vi "Instrumento_caracterizacion_3.vi"() -> ()   [LabVIEW 2009]
uses:
  <vilib>/Analysis/NI_AALBase.lvlib
panel:
  in  "Nombre de archivo":string="In1"
  in  "Activate switches 2":bool
  out "?":bool
  in  "Seleción método":bool
  in  "Ángulos de elementos ópticos:\nL2_in        L4_in     L4_out  P__out":dbl[](array[numeric])=[0.0, 0.0, 0.0, 0.0]
  in  "Amp vs ng":bool
  in  "fas vs ng":bool
  in  "Directorio scripts matlab 2":path=path "C:/Users/franjas/Documents/rutinas-calibracion-slm"
  in  "Exit live":bool
  in  "Capture":bool
  in  "stop":bool
  in  "File to load":path
  in  "File to save":path
  in  "VCD Properties":bool
  in  "Save properties":bool
  in  "Load properties":bool
  in  "Configurar para franjas":bool
  out "Histogram Graph":T1(graph)
  in  "Run live preview":bool
  out "Live Picture":picture
  out "Video formats":string[](array[string])
  out "Devices":string[](array[string])
  in  "ICImagingControl":refnum<k7>(container)
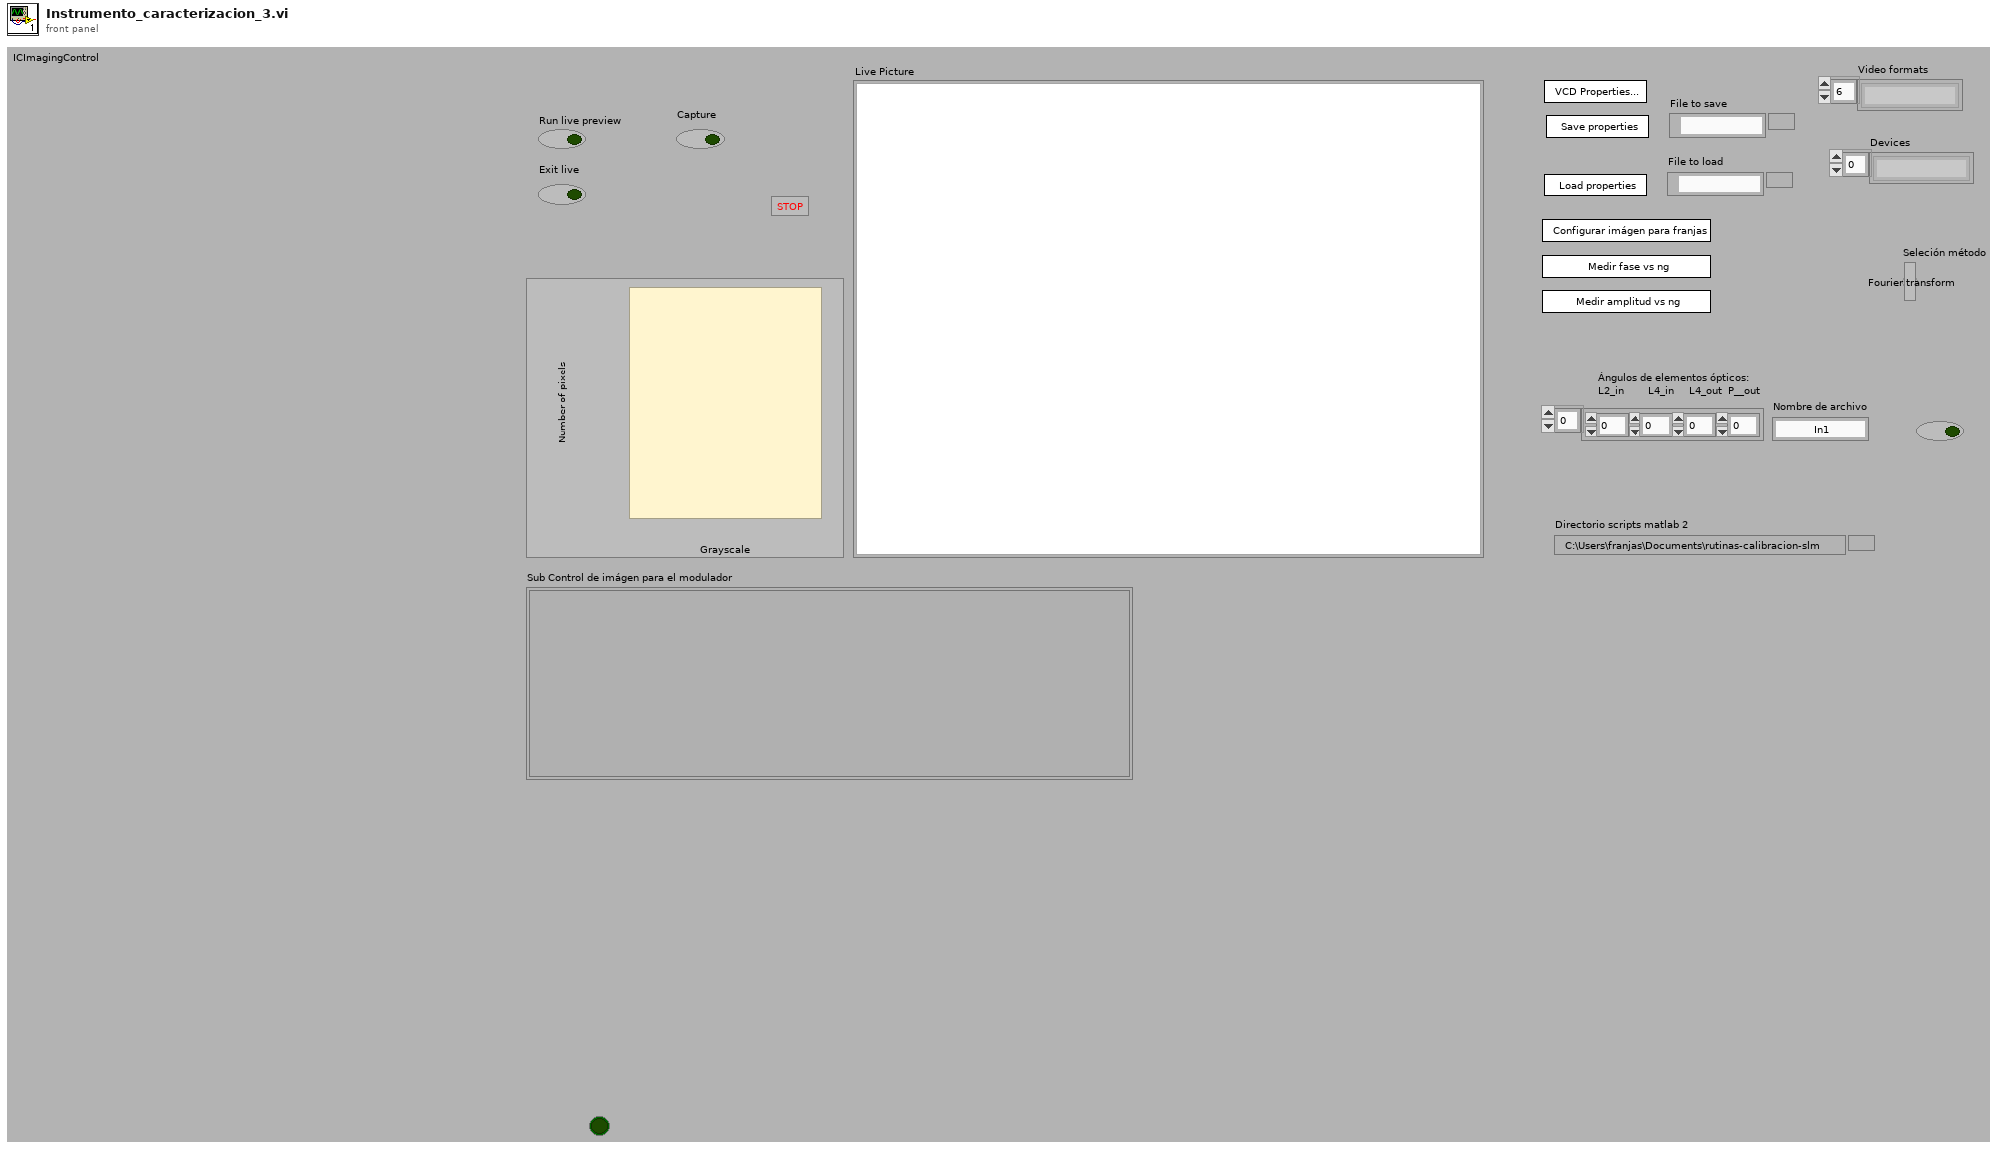
[diagram p1: front panel]
types:
  T1 = cluster{"X Values":dbl[], "Histogram: h(x)":i32[]}
  T2 = typedef "imagedata.ctl" = cluster{"image type":i32, "image depth":i32, "image":u8[], "mask":u8[], "colors":u32[], "Rectangle":cluster{"left":i16, "top":i16, "right":i16, "bottom":i16}}
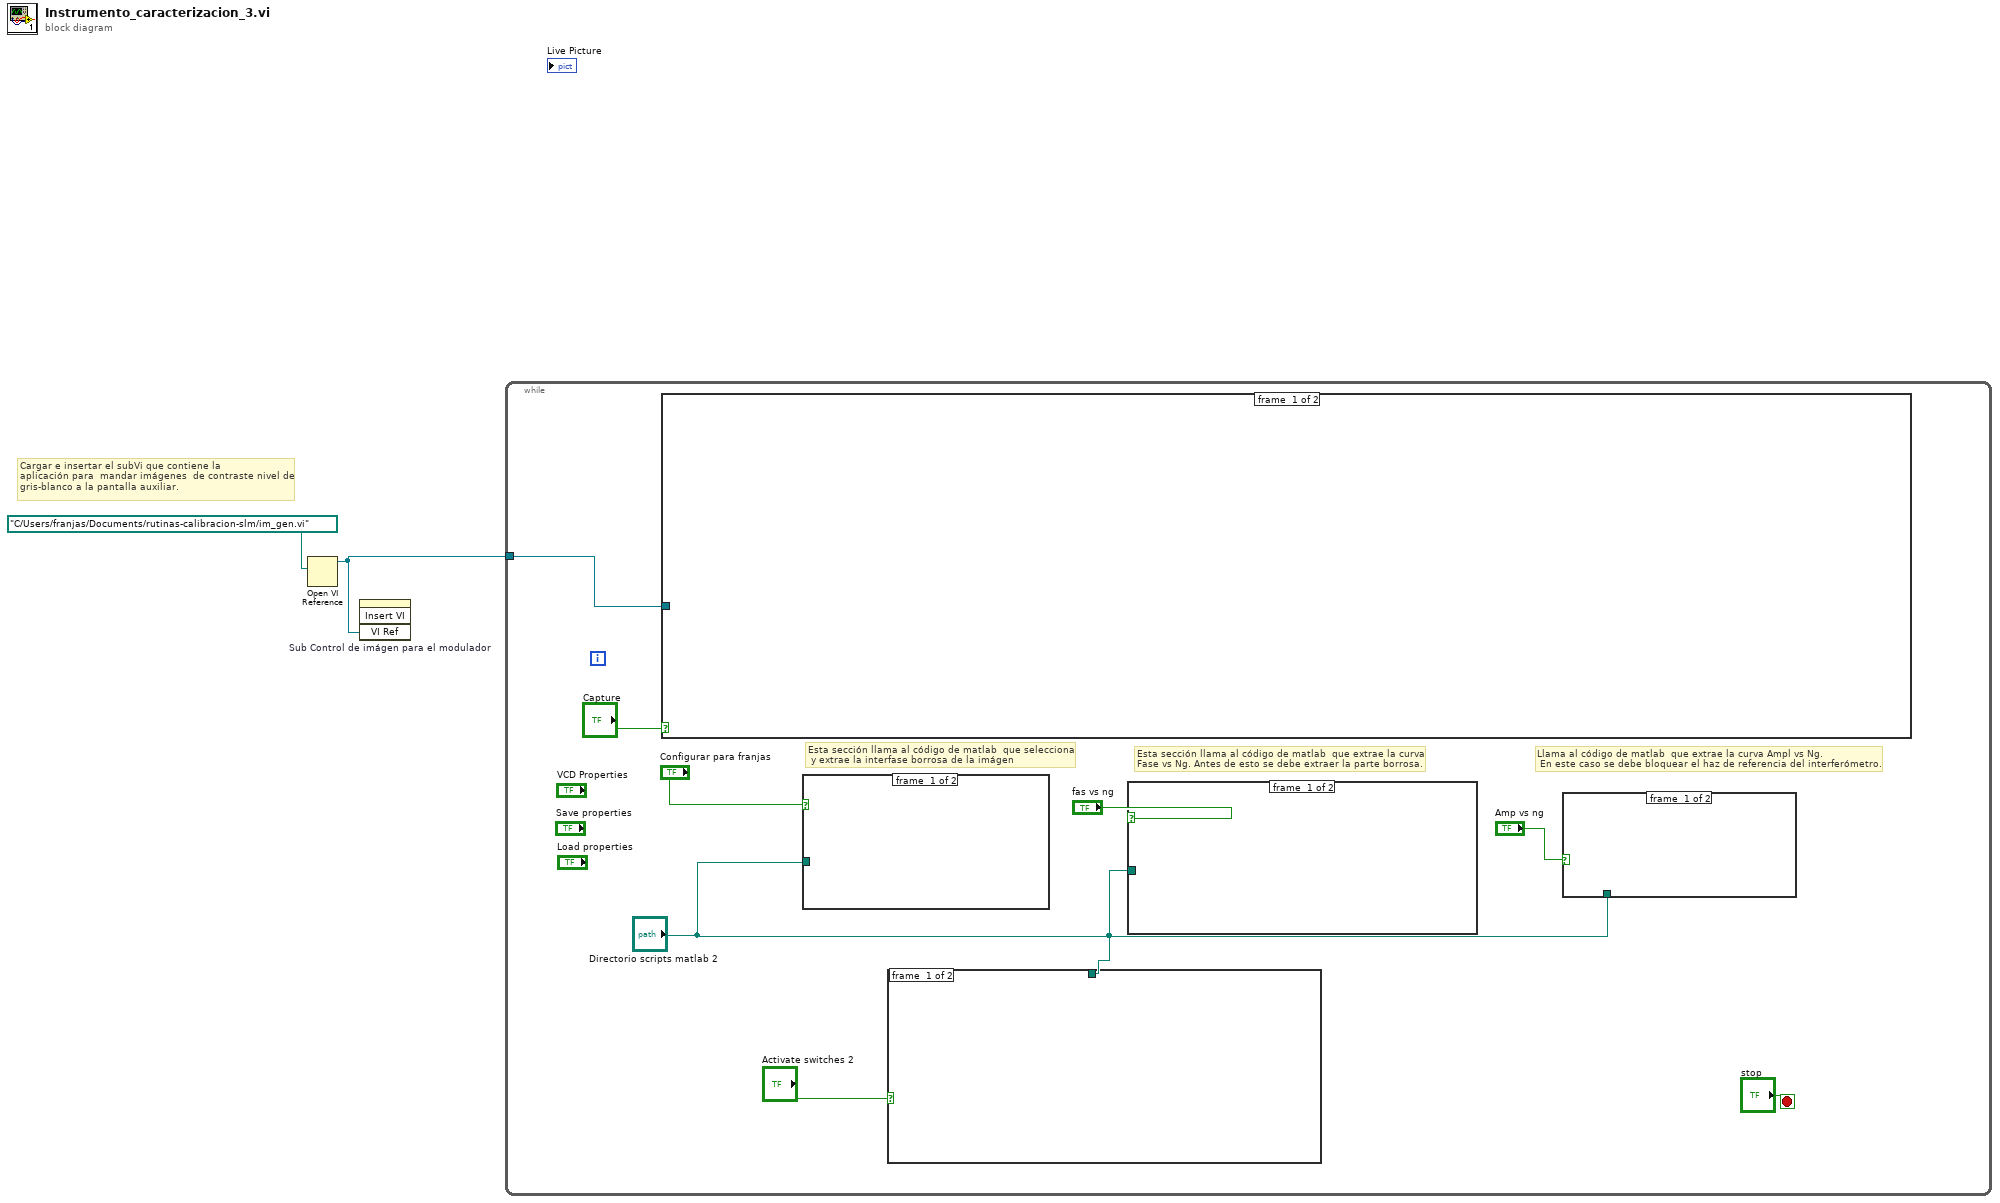
[diagram p0: block diagram]
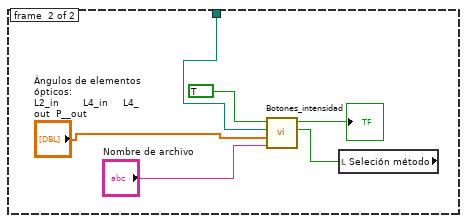
[diagram p2: hidden frame]
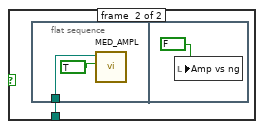
[diagram p3: hidden frame]
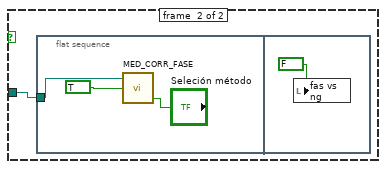
[diagram p4: hidden frame]
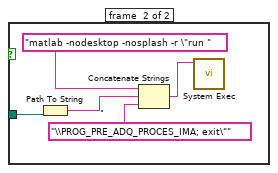
[diagram p5: hidden frame]
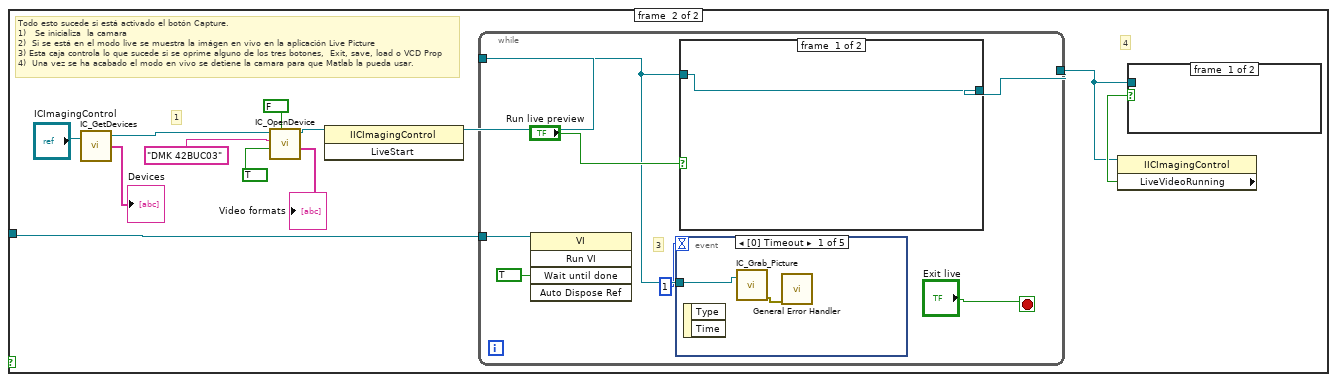
[diagram p6: hidden frame]
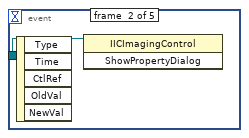
[diagram p7: hidden frame]
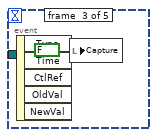
[diagram p8: hidden frame]
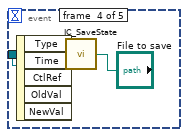
[diagram p9: hidden frame]
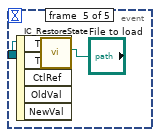
[diagram p10: hidden frame]
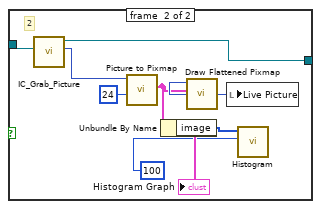
[diagram p11: hidden frame]
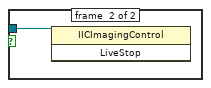
[diagram p12: hidden frame]
diagram:
  # "Cargar e insertar el subVi que contiene la \naplicación para  mandar imágenes  de contraste nivel de gris-blanco a la pantalla auxiliar."
  n1 = Open VI Reference(vi path=path "C:/Users/franjas/Documents/rutinas-calibracion-slm/im_gen.vi") -> (vi reference=w1:refnum<vi>)  [unwired: 5 in, 1 out]
  n2 = invoke on="Sub Control de imágen para el modulador" class="SubPanel" method="Insert VI"("VI Ref"=w1) -> ()  [unwired: 3 in, 4 out]
  n3 = while {
    tunnel: w1 -> [w7]
    stop <- "stop" stop-if-true
    # "Llama al código de matlab  que extrae la curva Ampl vs Ng.\n En este caso se debe bloquear el haz de referencia del interferómetro."
    # "Esta sección llama al código de matlab  que extrae la curva\nFase vs Ng. Antes de esto se debe extraer la parte borrosa."
    # "Esta sección llama al código de matlab  que selecciona\n y extrae la interfase borrosa de la imágen"
    n4 = case shown="True" "Capture" {
      tunnel: w7 -> [_ w31]
      frame #0 {
      }
      frame #1 {
        # "4"
        # "1"
        # "Todo esto sucede si está activado el botón Capture.  \n1)   Se inicializa  la camara \n2)  Si se está en el modo live se muestra la imágen en vivo en la aplicación Live Picture\n3) Esta caja controla lo que sucede si se oprime alguno de los tres botones,  Exit, save, load o VCD Prop\n4)  Una vez se ha acabado el modo en vivo se detiene la camara para que Matlab la pueda usar."
        n5 = call <userlib>:"IC_GetDevices.vi"("ICImagingControl In"="ICImagingControl") -> ("ICImagingControl Out"=w40:refnum<k7>, "Devices"=→"Devices":string[])  [unwired: 1 in, 1 out]
        n6 = call <userlib>:"IC_OpenDevice.vi"("Color"=FALSE, "Live"=TRUE, "Device"="DMK 42BUC03", "ICImagingControl In"=w40) -> ("VideoFormats"=→"Video formats":string[], "ICImagingControl Out"=w34:refnum<k7>)  [unwired: 2 in, 4 out]
        n7 = invoke class="IICImagingControl" method="LiveStart"(reference=w34) -> (reference out=w32:refnum<k7>)  [unwired: 2 in, 2 out]
        n8 = while {
          tunnel: w32 -> [w44]
          tunnel: [w49] -> w33
          tunnel: w31 -> [w46]
          stop <- "Exit live" stop-if-true
          # "3"
          n9 = invoke class="VI" method="Run VI"(reference=w46, "Wait until done"=TRUE ("Wait Until Done")) -> ()  [unwired: 3 in, 5 out]
          n10 = event shown="[0] Timeout" {
            selector: _ -> [_ _ _ _ _]
            dyn-events: _ -> [_ _ _ _ _]
            timeout: 1 -> [_ _ _ _ _]
            tunnel: w44 -> [w50 w52 _ w55 w57]
            event #0 {
              n11 = event-data() -> ()  [unwired: 1 in, 2 out]
              n12 = call <userlib>:"IC_Grab_Picture.vi"("ICImagingControl In"=w50) -> ("Error Out"=w51:errorcluster)  [unwired: 1 in, 3 out]
              n13 = call <vilib>:"General Error Handler.vi"("error in (no error)"=w51) -> ()  [unwired: 10 in, 5 out]
            }
            event #1 {
              n14 = event-data() -> ()  [unwired: 1 in, 5 out]
              n15 = invoke class="IICImagingControl" method="ShowPropertyDialog"(reference=w52) -> ()  [unwired: 2 in, 3 out]
            }
            event #2 {
              n16 = event-data() -> ()  [unwired: 1 in, 5 out]
              n17 = local write "Capture"(FALSE ("CApture")) -> ()
            }
            event #3 {
              n18 = event-data() -> ()  [unwired: 1 in, 5 out]
              n19 = call <userlib>:"IC_SaveState.vi"("file path"="File to save", "ICImagingControl In"=w55) -> ()  [unwired: 1 in, 2 out]
            }
            event #4 {
              n20 = event-data() -> ()  [unwired: 1 in, 5 out]
              n21 = call <userlib>:"IC_RestoreState.vi"("File Path"="File to load", "ICImagingControl"=w57) -> ()  [unwired: 2 in, 2 out]
            }
          }
          n22 = case shown="True" "Run live preview" {
            tunnel: w44 -> [w58 w64]
            tunnel: [w58 w59] -> w49
            frame #0 {
            }
            frame #1 {
              # "2"
              n23 = call <userlib>:"IC_Grab_Picture.vi"("ICImagingControl In"=w64) -> ("ICImagingControl Out"=w59:refnum<k7>, "Picture Out"=w67:picture)  [unwired: 1 in, 2 out]
              n24 = call <vilib>:"Picture to Pixmap.vi"("depth"=24, "picture"=w67) -> ("image data"=w63:T2)  [unwired: 8 in, 1 out]
              n25 = Unbundle By Name(w63) -> ("image"=w62:u8[])
              n26 = call <vilib>:"Draw Flattened Pixmap.vi"("image data"=w63) -> ("new picture"=w65:picture)  [unwired: 8 in]
              n27 = local write "Live Picture"(w65) -> ()
              n28 = call <vilib>:"Histogram.vi"("intervals"=100, "X"=w62) -> ("Histogram Graph"=→"Histogram Graph":T1)  [unwired: 6 in, 3 out]
            }
          }
        }
        n29 = property class="IICImagingControl"(reference=w33) -> ("LiveVideoRunning"=w35:bool)  [unwired: 1 in, 2 out]
        n30 = case shown="True" w35 {
          tunnel: w33 -> [_ w68]
          frame #0 {
          }
          frame #1 {
            n31 = invoke class="IICImagingControl" method="LiveStop"(reference=w68) -> ()  [unwired: 2 in, 3 out]
          }
        }
      }
    }
    n32 = case shown="True" "Configurar para franjas" {
      tunnel: "Directorio scripts matlab 2" -> [_ w26]
      frame #0 {
      }
      frame #1 {
        n33 = Path To String(path=w26) -> (string=w30:string)
        n34 = Concatenate Strings("matlab -nodesktop -nosplash -r \"run " ("command line"), w30, "\\PROG_PRE_ADQ_PROCES_IMA; exit\"" ("command line")) -> (w29:string)
        n35 = call <vilib>:"System Exec.vi"("command line"=w29) -> ()  [unwired: 7 in, 4 out]
      }
    }
    n36 = case shown="True" "Activate switches 2" {
      tunnel: "Directorio scripts matlab 2" -> [_ w16]
      frame #0 {
      }
      frame #1 {
        n37 = local read "Seleción método"() -> (w13:bool)
        n38 = call "Botones_intensidad.vi"("Seleción método"=w13, "String"="Nombre de archivo", "Array"="Ángulos de elementos ópticos:\nL2_in        L4_in     L4_out  P__out", "Directorio scripts matlab 2"=w16, "I1"=TRUE) -> (3:→"?":bool)  [unwired: 6 in]
      }
    }
    n39 = case shown="True" "fas vs ng" {
      tunnel: "Directorio scripts matlab 2" -> [_ w21]
      frame #0 {
      }
      frame #1 {
        n40 = flat-sequence {
          tunnel: w21 -> [w24]
          frame #0 {
            n41 = call "MED_CORR_FASE.vi"("Seleción método"="Seleción método", "Ejecucion"=TRUE ("Boolean"), "Directorio scripts matlab"=w24) -> ()
          }
          frame #1 {
            n42 = local write "fas vs ng"(FALSE ("fas vs ng")) -> ()
          }
        }
      }
    }
    n43 = case shown="True" "Amp vs ng" {
      tunnel: "Directorio scripts matlab 2" -> [_ w17]
      frame #0 {
      }
      frame #1 {
        n44 = flat-sequence {
          tunnel: w17 -> [w19]
          frame #0 {
            n45 = call "MED_AMPL.vi"("Boolean"=TRUE, "Directorio scripts matlab"=w19) -> ()  [unwired: 10 in]
          }
          frame #1 {
            n46 = local write "Amp vs ng"(FALSE ("Amp vs ng")) -> ()
          }
        }
      }
    }
  }
